vi "Init Loop.vi"(8 "error in (no error)":errorcluster, 11 "BluelinesRedlines in":refnum<class "BluelinesRedlines.lvclass">) -> (0 "error out":errorcluster, 3 "BluelinesRedlines out":refnum<class "BluelinesRedlines.lvclass">)   [LabVIEW 2020, in "VolatusGUIElements.lvlib" / "BluelinesRedlines.lvclass"]
uses:
  BluelinesRedlines.lvclass
  BluelinesRedlines.lvclass/BluelinesRedlines.ctl
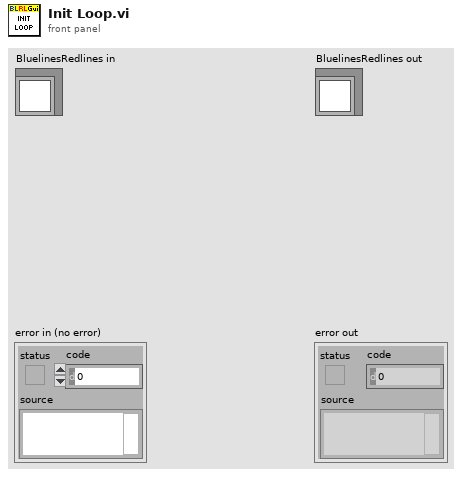
[diagram p1: front panel]
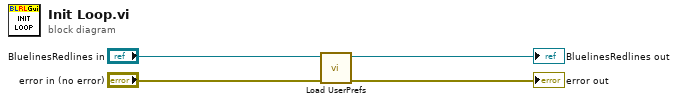
[diagram p0: block diagram]
diagram:
  n1 = call "Load UserPrefs.vi"("error in (no error)"="error in (no error)", "BluelinesRedlines in"="BluelinesRedlines in") -> ("error out"=→"error out":errorcluster, "BluelinesRedlines out"=→"BluelinesRedlines out":refnum<class "BluelinesRedlines.lvclass">)  [unwired: 8 in]
